vi "GLdrv_TRANS_OPEN.vi"(0 "Connection ID":T1, 11 "error in (no error)":errorcluster) -> (4 "Connection ID Out":T1, 6 "Error Code":i16, 8 "ID out":i32, 15 "error out":errorcluster)   [LabVIEW 2017, in "GL860_Driver.lvlib"]
doc: "SOURceで設定されたファイルに対してオープン処理を行います\nレスポンスとして3バイトのバイナリが送信されます\n[1バイト目] ID番号\n[2バイト目] 未使用\n[3バイト目] \n76543210\n|||||||+-1ならオープン失敗\n+++++++--未使用"
uses:
  GL860_Driver.lvlib
  ConnectionID.ctl
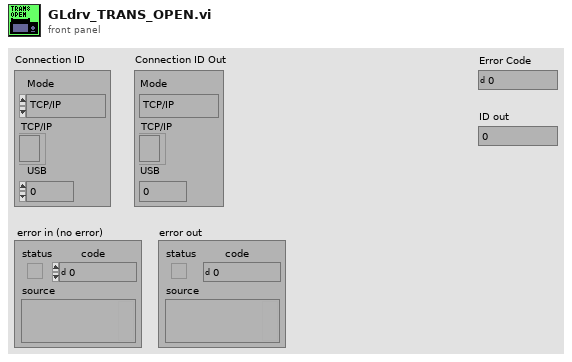
[diagram p1: front panel]
types:
  T1 = typedef "ConnectionID.ctl" = cluster{"Mode":enum16{"TCP/IP", "USB"}, "TCP/IP":refnum<k5>, "USB":i32}
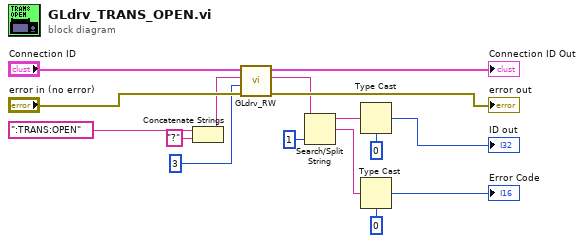
[diagram p0: block diagram]
diagram:
  n1 = Concatenate Strings(":TRANS:OPEN" ("Command"), "?" ("string")) -> (w10:string)
  n2 = call "GLdrv_RW.vi"("error in (no error)"="error in (no error)", "Count(0:[CR+LF])"=u32 3, "data in"=w10, "Connection ID"="Connection ID") -> ("error out"=→"error out":errorcluster, "data out"=w4:string, "Connection ID Out"=→"Connection ID Out":T1)  [unwired: 3 in, 2 out]
  n3 = Search/Split String(string=w4, offset (0)=1) -> (substring before match=w7:string, match + rest of string=w6:string)  [unwired: 2 out]
  n4 = Type Cast(type=u8 0 ("Status"), x=w7) -> (*(type *) &x=→"ID out":u8)
  n5 = Type Cast(type=i16 0 ("Status"), x=w6) -> (*(type *) &x=→"Error Code":i16)
